vi "Acknowledge Post Process.vi"(8 "error in (no error)":errorcluster, 10 "Ack Result":refnum<class "Acquired Result.lvclass">, 11 "Measure Controller in":refnum<class "Process Controller.lvclass">) -> (0 "error out":errorcluster, 3 "Measure Controller out":refnum<class "Process Controller.lvclass">)   [LabVIEW 2016, in "Process Controller.lvclass"]
uses:
  Process Controller.lvclass
  Results/Acquired Result/Acquired Result.lvclass
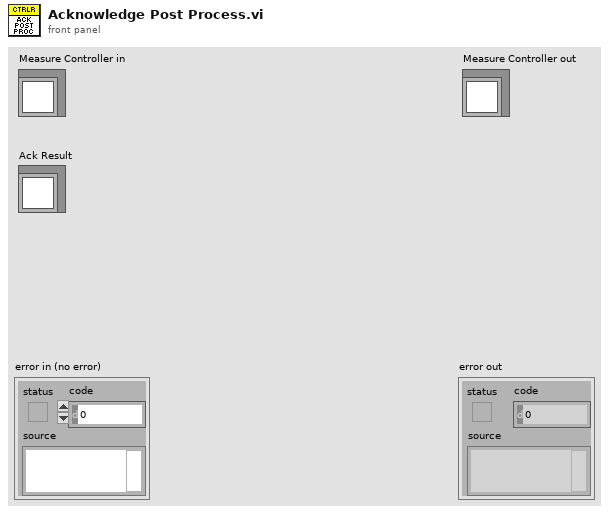
[diagram p1: front panel]
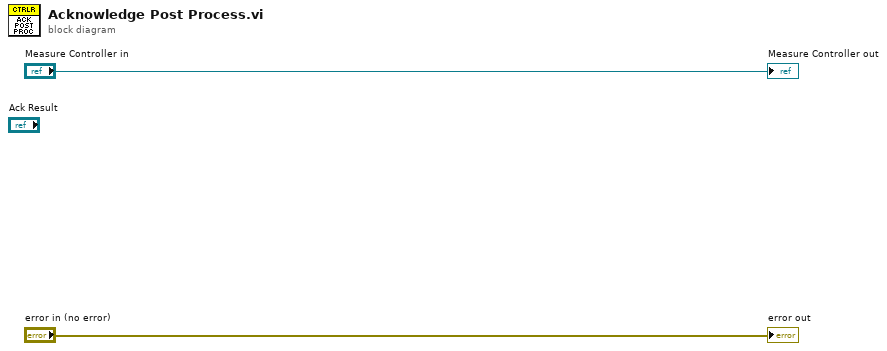
[diagram p0: block diagram]
diagram:
  "error out" <- "error in (no error)"
  "Measure Controller out" <- "Measure Controller in"
